vi "Save Current Fov.vi"(7 "Max Zoom":i32, 8 "error in":errorcluster, 10 "Current FOV":cluster{"Width [um]":dbl, "Height [um]":dbl}={"Width [um]"=400.0, "Height [um]"=400.0}, 11 "Current Zoom":i32) -> (0 "error out":errorcluster, 2 "Updated":bool)   [LabVIEW 2012, in "Sciscan Scope Daemon.lvlib"]
uses:
  Sciscan Scope Daemon.lvlib
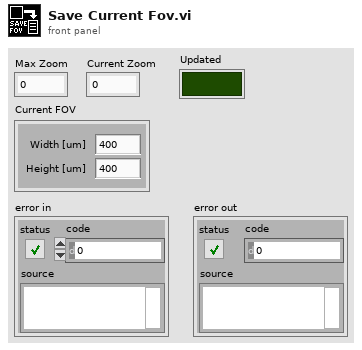
[diagram p1: front panel]
types:
  T1 = enum16{"Left Button", "Center Button", "Right Button", "Window Close"}
  T2 = enum16{"open", "replace", "create", "open or create", "replace or create", "replace or create with confirmation"}
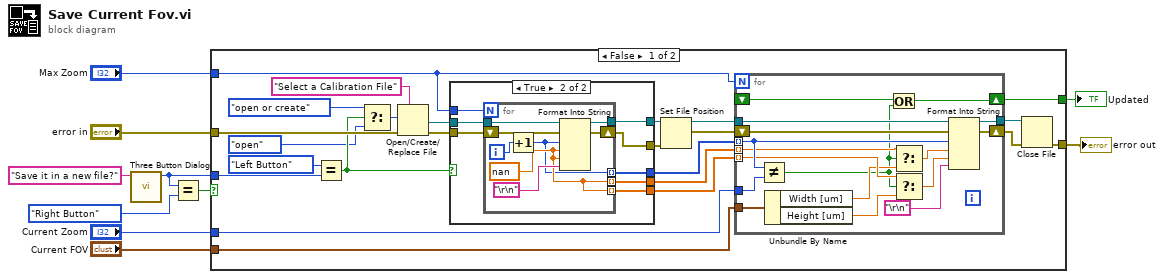
[diagram p0: block diagram]
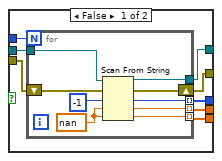
[diagram p2: hidden frame]
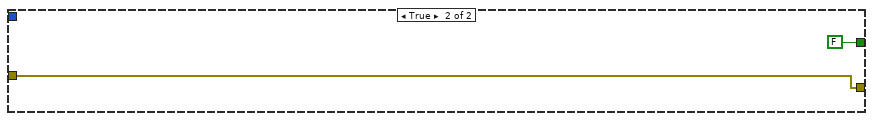
[diagram p3: hidden frame]
diagram:
  n1 = call <vilib>:"Three Button Dialog.vi"("message"="Save it in a new file?") -> ("Which Button?"=w6:T1)  [unwired: 10 in]
  n2 = Equal?(x=w6, y=T1."Right Button") -> (x = y?=w7:bool)
  n3 = case shown="False" w7 {
    tunnel: "error in" -> [w34 w85]
    tunnel: w6 -> [w26 _]
    tunnel: [w16 FALSE] -> w5
    tunnel: [w15 w85] -> w4
    tunnel: "Current Zoom" -> [w14 _]
    tunnel: "Current FOV" -> [w13 _]
    tunnel: "Max Zoom" -> [w11 _]
    frame False {
      n4 = Equal?(x=T1."Left Button" ("Which Button?"), y=w26) -> (x = y?=w31:bool)
      n5 = Select(t=T2."open or create" ("operation (0:open)"), s=w31, f=T2."open" ("operation (0:open)")) -> (s? t:f=w28:T2)
      n6 = Open/Create/Replace File(error in=w34, prompt="Select a Calibration File", operation (0:open)=w28) -> (refnum out=w27:refnum<file>, error out=w33:errorcluster)  [unwired: 3 in, 1 out]
      n7 = case shown="True" w31 {
        tunnel: w33 -> [w59 w76]
        tunnel: w27 -> [w58 w75]
        tunnel: w11 -> [w57 w74]
        tunnel: [w56 w73] -> w24
        tunnel: [w55 w72] -> w25
        tunnel: [w54 w71] -> w21
        tunnel: [w53 w70] -> w20
        tunnel: [w52 w69] -> w19
        frame False {
          n8 = for {
            N: w57 -> [_]
            tunnel: [w66] -> w56
            shift-right: [w64] -> w55
            shift-left: w59 -> [w65]
            tunnel: [w63] -> w52 mode=indexing
            tunnel: [w62] -> w53 mode=indexing
            tunnel: [w61] -> w54 mode=indexing
            tunnel: w58 -> [w60]
            w67 = nan ("input 3")
            n9 = Scan From String(w60, w65, default 1=-1, default 2=w67, default 3=w67) -> (w66:refnum<file>, w64:errorcluster, output 1=w61:i32, output 2=w62:dbl, output 3=w63:dbl)  [unwired: 1 in]
          }
        }
        frame True {
          n10 = for {
            N: w74 -> [_]
            tunnel: [w83] -> w73
            shift-right: [w84] -> w72
            shift-left: w76 -> [w82]
            tunnel: [w77] -> w71 mode=indexing
            tunnel: [w79] -> w70 mode=indexing
            tunnel: [w79] -> w69 mode=indexing
            tunnel: w75 -> [w78]
            i -> [w80]
            w79 = nan ("input 2")
            n11 = Increment(x=w80) -> (x+1=w77:i32)
            n12 = Format Into String(initial string=w78, error in=w82, w77, w79, w79, "\r\n") -> (resulting string=w83:refnum<file>, error out=w84:errorcluster)  [unwired: 1 in]
          }
        }
      }
      n13 = Set File Position(refnum=w24, error in=w25) -> (refnum out=w22:refnum<file>, error out=w23:errorcluster)  [unwired: 2 in]
      n14 = for {
        N: w11 -> [_]
        tunnel: w22 -> [w49]
        tunnel: [w50] -> w17
        shift-right: [w51] -> w18
        shift-left: w23 -> [w48]
        tunnel: w21 -> [w46] mode=indexing
        tunnel: w20 -> [w38] mode=indexing
        tunnel: w19 -> [w41] mode=indexing
        tunnel: w13 -> [w44]
        tunnel: w14 -> [w45]
        shift-right: [w37] -> w16
        shift-left: _ -> [w35]
        n15 = Not Equal?(x=w46, y=w45) -> (x != y?=w36:bool)
        n16 = Unbundle By Name(w44) -> ("Width [um]"=w39:dbl, "Height [um]"=w40:dbl)
        n17 = Or(x=w35, y=w36) -> (x .or. y?=w37:bool)
        n18 = Select(t=w38, s=w36, f=w39) -> (s? t:f=w43:dbl)
        n19 = Select(t=w41, s=w36, f=w40) -> (s? t:f=w42:dbl)
        n20 = Format Into String(initial string=w49, error in=w48, w46, w43, w42, "\r\n") -> (resulting string=w50:refnum<file>, error out=w51:errorcluster)  [unwired: 1 in]
      }
      n21 = Close File(refnum=w17, error in=w18) -> (error out=w15:errorcluster)  [unwired: 1 out]
    }
    frame True {
    }
  }
  "Updated" <- w5
  "error out" <- w4
